vi "draw_cross_section.vi"(7 "highlight?":bool, 8 "error in (no error)":errorcluster, 9 "depth":dbl[unit], 10 "Image.lvclass":refnum<class "Image.lvclass">, 11 "RoiEllipsoid in":refnum<class "RoiEllipsoid.lvclass">=refnum) -> (0 "error out":errorcluster, 3 "RoiEllipsoid out":refnum<class "RoiEllipsoid.lvclass">)   [LabVIEW 2010, in "RoiEllipsoid.lvclass"]
uses:
  RoiEllipsoid.lvclass
  common/classes/Image/Image/Image.lvclass
  common/classes/Box/Box/Box.lvclass
  common/classes/SpaceVector/SpaceVector/SpaceVector.lvclass
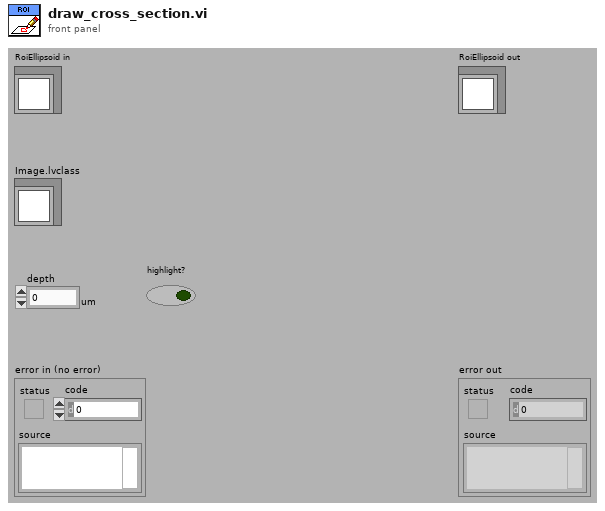
[diagram p1: front panel]
types:
  T1 = cluster{"[0]":i32, "[1]":i32, "[2]":i32, "[3]":i32}
  T2 = typedef "IMAQ Image.ctl" = refnum<image>
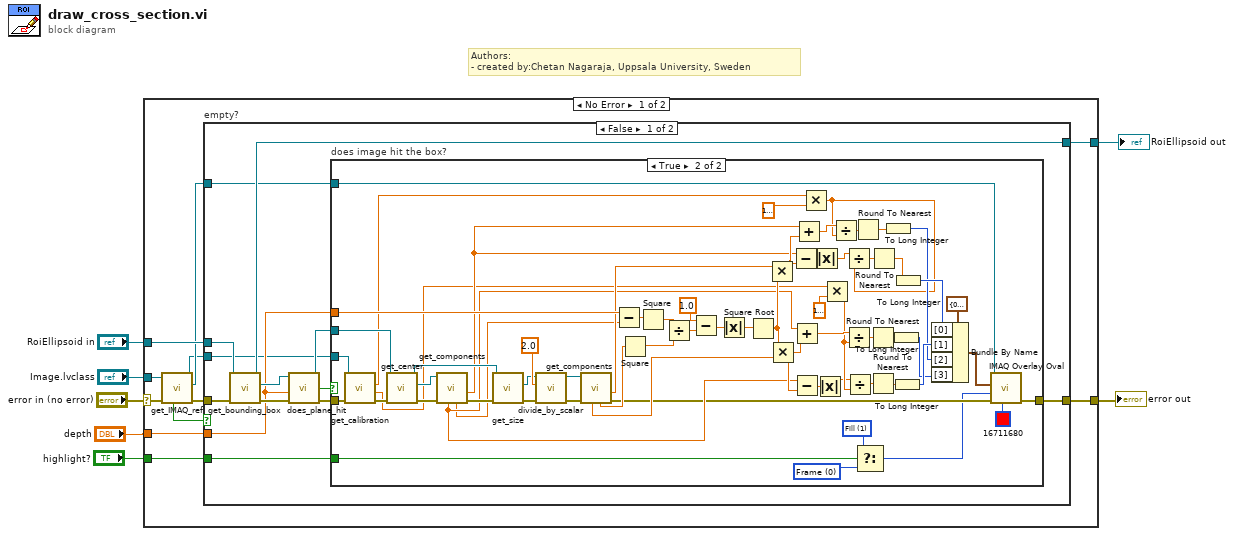
[diagram p0: block diagram]
diagram:
  # "Authors: \n- created by:Chetan Nagaraja, Uppsala University, Sweden"
  n1 = case shown="No Error" "error in (no error)" {
    selector: "error in (no error)" -> [w14 w100]
    tunnel: [w16 w100] -> w3
    tunnel: [w17 w99] -> w2
    tunnel: "RoiEllipsoid in" -> [w18 w99]
    tunnel: "depth" -> [w15 _]
    tunnel: "Image.lvclass" -> [w11 _]
    tunnel: "highlight?" -> [w8 _]
    frame No Error {
      n2 = call-dynamic "get_IMAQ_ref.vi"("error in (no error)"=w14, "Image.lvclass in"=w11) -> ("error out"=w13:errorcluster, "Image"=w10:T2, "Image.lvclass out"=w9:refnum<class "Image.lvclass">, "empty?"=w12:bool)  [unwired: 5 in, 1 out]
      n3 = case "empty?" shown="False" w12 {
        tunnel: w13 -> [w30 w97]
        tunnel: w18 -> [w28 w98]
        tunnel: [w27 w98] -> w17
        tunnel: [w24 w97] -> w16
        tunnel: w15 -> [w22 _]
        tunnel: w10 -> [w21 _]
        tunnel: w9 -> [w20 _]
        tunnel: w8 -> [w19 _]
        frame False {
          n4 = call-dynamic "get_bounding_box.vi"("error in (no error)"=w30, "RoiGeneric in"=w28) -> ("error out"=w29:errorcluster, "Box.lvclass"=w26:refnum<class "Box.lvclass">, "RoiGeneric out"=w27:refnum<class "RoiEllipsoid.lvclass">)  [unwired: 7 in]
          n5 = call "does_plane_hit.vi"("error in (no error)"=w29, "depth"=w22, "Box in"=w26) -> ("error out"=w25:errorcluster, "is inside?"=w31:bool, "Box out"=w23:refnum<class "Box.lvclass">)  [unwired: 6 in]
          n6 = case "does image hit the box?" shown="True" w31 {
            tunnel: w25 -> [w32 w53]
            tunnel: [w32 w58] -> w24
            tunnel: w23 -> [_ w96]
            tunnel: w22 -> [_ w91]
            tunnel: w21 -> [_ w54]
            tunnel: w20 -> [_ w51]
            tunnel: w19 -> [_ w36]
            frame False {
            }
            frame True {
              w34 = u32 1 items=["Frame", "Fill"] ("Drawing Mode (Frame)")
              w35 = u32 0 items=["Frame", "Fill"] ("Drawing Mode (Frame)")
              n7 = call "get_calibration.vi"("error in (no error)"=w53, "Image.lvclass in"=w51) -> ("error out"=w52:errorcluster, "y"=w42:dbl, "x"=w49:dbl)  [unwired: 4 in, 3 out]
              n8 = call "get_center.vi"("error in (no error)"=w52, "Box in"=w96) -> ("error out"=w93:errorcluster, "center"=w94:refnum<class "SpaceVector.lvclass">, "Box out"=w95:refnum<class "Box.lvclass">)  [unwired: 7 in]
              n9 = call "get_components.vi"("error in (no error)"=w93, "SpaceVector in"=w94) -> ("error out"=w92:errorcluster, "x"=w75:dbl[unit], "z"=w55:dbl[unit], "y"=w69:dbl[unit])  [unwired: 4 in, 2 out]
              n10 = call "get_size.vi"("error in (no error)"=w92, "Box in"=w95) -> ("error out"=w80:errorcluster, "size"=w77:refnum<class "SpaceVector.lvclass">)  [unwired: 7 in, 1 out]
              n11 = call "divide_by_scalar.vi"("error in (no error)"=w80, "divisor"=2.0, "SpaceVector in"=w77) -> ("error out"=w79:errorcluster, "SpaceVector out"=w76:refnum<class "SpaceVector.lvclass">)  [unwired: 7 in]
              n12 = call "get_components.vi"("error in (no error)"=w79, "SpaceVector in"=w76) -> ("error out"=w57:errorcluster, "x"=w84:dbl[unit], "z"=w89:dbl[unit], "y"=w83:dbl[unit])  [unwired: 4 in, 2 out]
              n13 = Subtract(x=w91, y=w55) -> (x-y=w90:dbl[unit])
              n14 = Square(x=w89) -> (x^2=w87:dbl[unit])
              n15 = Square(x=w90) -> (x^2=w88:dbl[unit])
              n16 = Divide(x=w88, y=w87) -> (x/y=w86:dbl)
              n17 = Subtract(x=1.0, y=w86) -> (x-y=w72:dbl)
              n18 = Absolute Value(x=w72) -> (abs(x)=w73:dbl)
              n19 = Square Root(x=w73) -> (sqrt(x)=w82:dbl)
              n20 = Multiply(x=w84, y=w82) -> (x*y=w81:dbl[unit])
              n21 = Multiply(x=w82, y=w83) -> (x*y=w70:dbl[unit])
              n22 = Subtract(x=w75, y=w81) -> (x-y=w74:dbl[unit])
              n23 = Add(x=w69, y=w70) -> (x+y=w41:dbl[unit])
              n24 = Subtract(x=w69, y=w70) -> (x-y=w71:dbl[unit])
              n25 = Add(x=w75, y=w81) -> (x+y=w47:dbl[unit])
              n26 = Multiply(x=w49, y=dbl[unit] 1e-06 ("element")) -> (x*y=w45:dbl[unit])
              n27 = Absolute Value(x=w74) -> (abs(x)=w44:dbl[unit])
              n28 = Absolute Value(x=w71) -> (abs(x)=w37:dbl[unit])
              n29 = Multiply(x=w42, y=dbl[unit] 1e-06 ("element")) -> (x*y=w39:dbl[unit])
              n30 = Divide(x=w47, y=w45) -> (x/y=w48:dbl)
              n31 = Divide(x=w44, y=w45) -> (x/y=w46:dbl)
              n32 = Divide(x=w41, y=w39) -> (x/y=w40:dbl)
              n33 = Divide(x=w37, y=w39) -> (x/y=w38:dbl)
              n34 = Round To Nearest(number=w48) -> (nearest integer value=w67:dbl)
              n35 = Select(t=w34, s=w36, f=w35) -> (s? t:f=w33:u32)
              n36 = Round To Nearest(number=w40) -> (nearest integer value=w65:dbl)
              n37 = Round To Nearest(number=w38) -> (nearest integer value=w63:dbl)
              n38 = Round To Nearest(number=w46) -> (nearest integer value=w66:dbl)
              n39 = To Long Integer(number=w67) -> (32bit integer=w61:i32)
              n40 = To Long Integer(number=w65) -> (32bit integer=w60:i32)
              n41 = To Long Integer(number=w63) -> (32bit integer=w62:i32)
              n42 = To Long Integer(number=w66) -> (32bit integer=w64:i32)
              n43 = Bundle By Name(cluster=T1 {"[0]"=0, "[1]"=0, "[2]"=0, "[3]"=0}, "[0]"=w64, "[1]"=w62, "[2]"=w61, "[3]"=w60) -> (w59:T1)
              n44 = call "IMAQ Overlay Oval"("Color"=u32 16711680, "error in (no error)"=w57, "Drawing Mode (Frame)"=w33, "Bounding Rectangle"=w59, "Image"=w54) -> ("error out"=w58:errorcluster)  [unwired: 5 in, 1 out]
            }
          }
        }
        frame True {
        }
      }
    }
    frame Error {
    }
  }
  "error out" <- w3
  "RoiEllipsoid out" <- w2
